vi "VI Server Launcher.vi"() -> ()   [LabVIEW 2021]
uses:
  <vilib>/Utility/LVLibp/NI_PackedLibraryUtility.lvlib
panel:
  out "error out":errorcluster
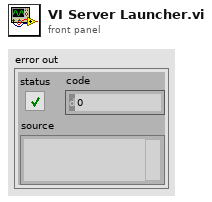
[diagram p1: front panel]
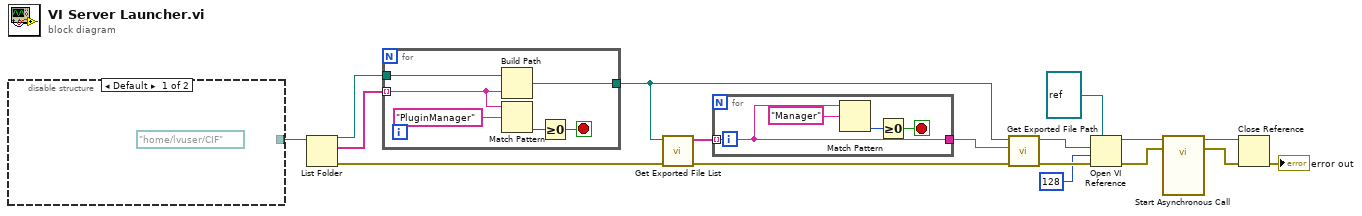
[diagram p0: block diagram]
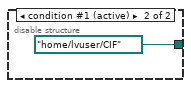
[diagram p2: hidden frame]
diagram:
  n1 = disable-structure shown="Default" {
    disable-tunnel: [_ path "/home/lvuser/CIF" ("packed library path")] -> w15
    frame condition #0 {
      (unwired) path "/home/lvuser/CIF" ("packed library path")
    }
    frame condition #1 (active) {
    }
  }
  n2 = List Folder(path=w15) -> (path out=w12:path, filenames=w13:string[], error out=w14:errorcluster)  [unwired: 3 in, 1 out]
  n3 = for {
    tunnel: w13 -> [w19] mode=indexing
    tunnel: [w20] -> w1
    tunnel: w12 -> [w21]
    stop <- w23 stop-if-true
    n4 = Build Path(base path=w21, name or relative path=w19) -> (appended path=w20:path)
    n5 = Match Pattern(string=w19, regular expression="PluginManager") -> (offset past match=w24:i32)  [unwired: 1 in, 3 out]
    n6 = Greater Or Equal To 0?(x=w24) -> (x >= 0?=w23:bool)
  }
  n7 = call <vilib>:"Get Exported File List.vi"("error in (no error)"=w14, "packed library path"=w1) -> ("error out"=w16:errorcluster, "qualified names"=w17:string[])  [unwired: 7 in, 1 out]
  n8 = for {
    tunnel: w17 -> [w25] mode=indexing
    tunnel: [w25] -> w2
    stop <- w27 stop-if-true
    n9 = Match Pattern(string=w25, regular expression="Manager") -> (offset past match=w28:i32)  [unwired: 1 in, 3 out]
    n10 = Greater Or Equal To 0?(x=w28) -> (x >= 0?=w27:bool)
  }
  n11 = call <vilib>:"Get Exported File Path.vi"("error in (no error)"=w16, "qualified name"=w2, "packed library path"=w1) -> ("error out"=w10:errorcluster, "path"=w11:path)  [unwired: 7 in]
  n12 = Open VI Reference(type specifier VI Refnum (for type only)=refnum<vi> refnum, vi path=w11, options=128, error in (no error)=w10) -> (vi reference=w7:refnum<vi>, error out=w6:errorcluster)  [unwired: 2 in]
  n13 = call-by-ref "Start Asynchronous Call"(reference=w7, error in=w6) -> (reference out=w5:refnum<vi>, error out=w4:errorcluster)  [unwired: 12 in]
  n14 = Close Reference(reference=w5, error in (no error)=w4) -> (error out=→"error out":errorcluster)
